vi "Laser_Controller.vi"() -> ()   [LabVIEW 2009]
panel:
  out "Init Error":u32
  out "Intensity (a.u.)":dbl
  out "Close Error Number":u32 format="%.0x"
  in  "PCI Can":bool=TRUE
  out "Excitation":bool
  out "Detector1":bool
  out "Detector2":bool
  out "Intensity (a.u.)":dbl=1.0 format="%.02f"
  in  "Laser(unused)":dbl(slide) scale=0.0..100.0
  in  "?":i16(slide) min=-100 max=100 step=1 scale=-100.0..100.0
  in  "Laser 637 nm (red)":dbl(slide) scale=0.0..100.0
  in  "?":i16(slide) min=-100 max=100 step=1 scale=-100.0..100.0
  in  "Laser 532 nm (green)":dbl(slide) scale=0.0..100.0
  in  "?":i16(slide) min=-100 max=100 step=1 scale=-100.0..100.0
  in  "Laser 470 nm (blue)":dbl(slide) scale=0.0..100.0
  in  "?":i16(slide) min=-100 max=100 step=1 scale=-100.0..100.0
  out "Laser 5 pos.":u16
  out "Laser 6 pos.":u16
  out "Laser 7 pos.":u16
  out "Laser 8 pos.":u16
  out "Laser 4 pos.":u16
  out "Laser 3 pos.":u16
  out "Laser 2 pos.":u16
  out "Laser 1 pos.":u16
  in  "stop":bool
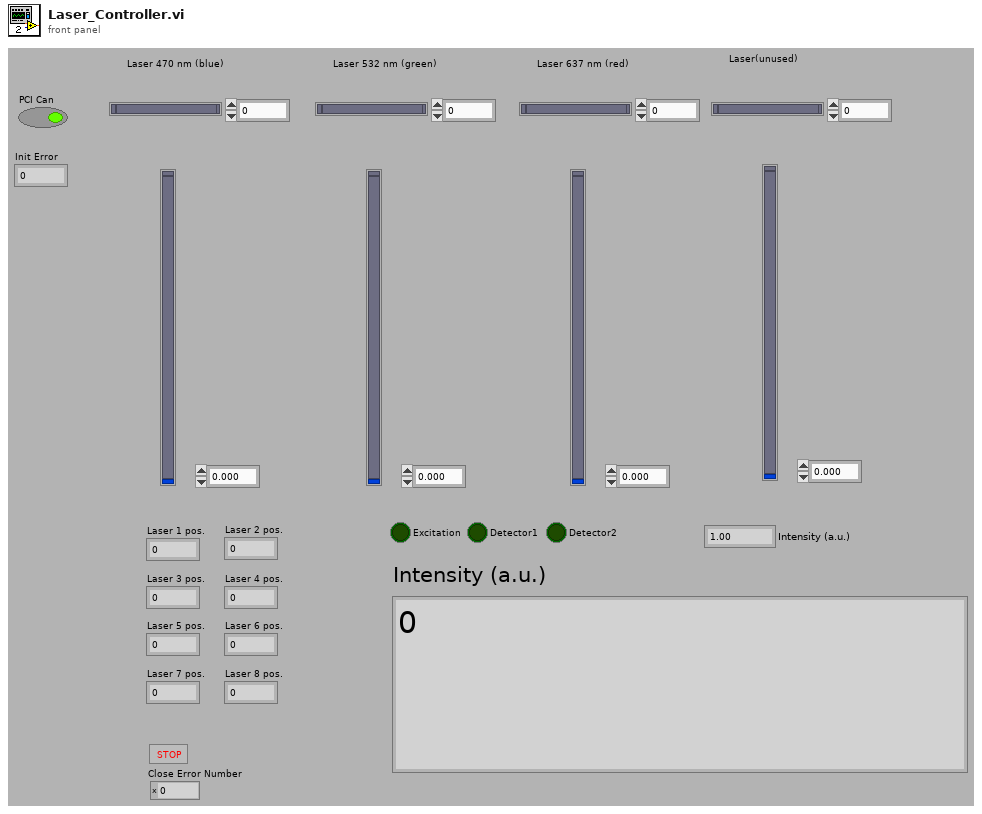
[diagram p1: front panel]
types:
  T1 = enum16{"CAN_Baud_1M", "CAN_BAUD_500K", "CAN_BAUD_250K", "CAN_BAUD_125K", "CAN_BAUD_100K", "CAN_BAUD_50K", "CAN_BAUD_20K", "CAN_BAUD_10K", "CAN_BAUD_5K", "User"}
  T2 = enum8{"STD, NO RTR", "STD,RTR", "XTD, NO RTR", "XTD, RTR"}
  T3 = cluster{"ID":u32, "MSG type":enum8{"STD, NO RTR", "STD,RTR", "XTD, NO RTR", "XTD, RTR"}, "LEN":u8, "DATA":u8[]}
  T4 = cluster{"x":u32, "MSG type":enum8{"STD, NO RTR", "STD,RTR", "XTD, NO RTR", "XTD, RTR"}, "LEN 3":u8, u8[]}
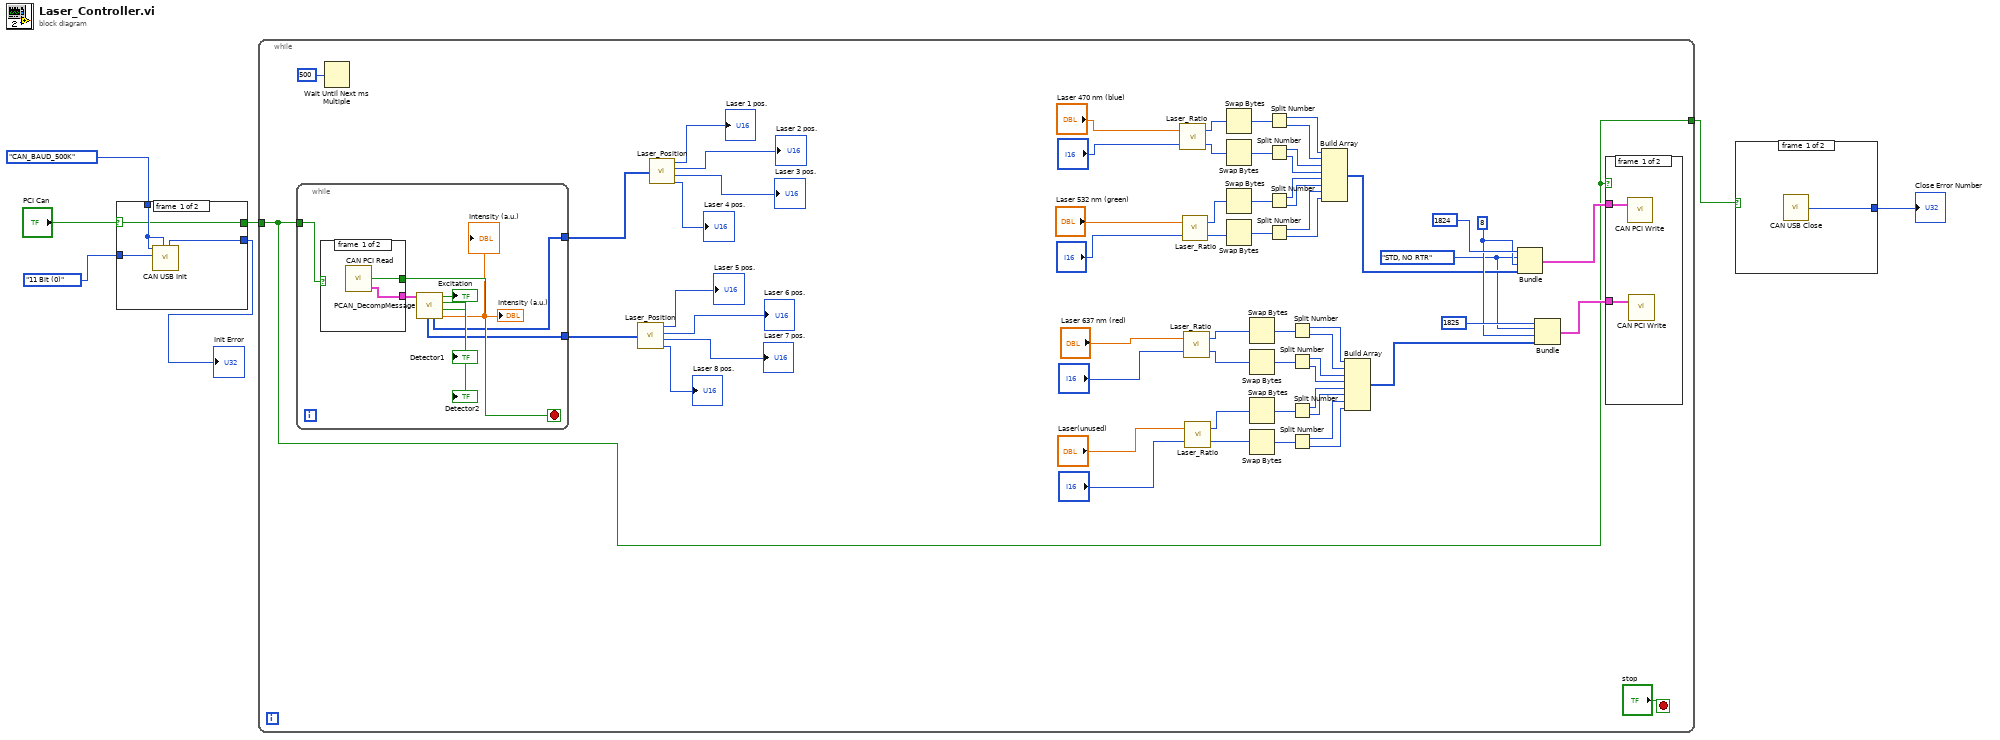
[diagram p0: block diagram]
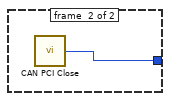
[diagram p2: hidden frame]
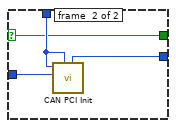
[diagram p3: hidden frame]
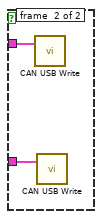
[diagram p4: hidden frame]
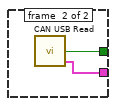
[diagram p5: hidden frame]
diagram:
  n1 = case shown="False" "PCI Can" {
    selector: "PCI Can" -> [w9 w13]
    tunnel: enum16{"11 Bit (0)", "29/11 Bit (1)"}."11 Bit (0)" ("CAN Msg Type") -> [w11 w15]
    tunnel: T1."CAN_BAUD_500K" ("BTR0BTR1") -> [w10 w14]
    tunnel: [w9 w13] -> w4
    tunnel: [w8 w12] -> w1
    frame #0 {
      n2 = call "CAN USB Init.vi"("BTR0BTR1(User)"=w10, "CAN Msg Type"=w11, "BTR0BTR1"=w10) -> ("Error Number"=w8:u32)  [unwired: 6 in, 2 out]
    }
    frame #1 {
      n3 = call "CAN PCI Init.vi"("BTR0BTR1(User)"=w14, "CAN Msg Type"=w15, "BTR0BTR1"=w14) -> ("Error Number"=w12:u32)  [unwired: 6 in, 2 out]
    }
  }
  "Init Error" <- w1
  n4 = while {
    tunnel: w4 -> [w16]
    tunnel: [w16] -> w3
    stop <- "stop" stop-if-true
    w38 = T2."STD, NO RTR" ("MSG type")
    w70 = u8 8 ("LEN 3")
    n5 = while {
      tunnel: w16 -> [w83]
      tunnel: [w82] -> w18
      tunnel: [w81] -> w17
      stop <- w89 stop-if-true
      n6 = case shown="True" w83 {
        tunnel: [w91 w93] -> w89
        tunnel: [w90 w92] -> w88
        frame #0 {
          n7 = call "CAN PCI Read.vi"() -> ("RcvQueueEmpty"=w91:bool, "CAN_Message out"=w90:T3)  [unwired: 1 in, 1 out]
        }
        frame #1 {
          n8 = call "CAN USB Read.vi"() -> ("RcvQueueEmpty"=w93:bool, "CAN_Message out"=w92:T3)  [unwired: 1 in, 1 out]
        }
      }
      n9 = call "PCAN_DecompMessage.vi"("CAN_Message out"=w88) -> ("Intensity (a.u.)"=→"Intensity (a.u.)" →"Intensity (a.u.)":dbl, "Detector2 Shutter Open?"=→"Detector2":bool, "Detector1 Shutter Open?"=→"Detector1":bool, "Excitation Shutter Open?"=→"Excitation":bool, "Laser 1-4"=w82:u8[], "Laser 5-8"=w81:u8[])  [unwired: 5 in]
    }
    n10 = Wait Until Next ms Multiple(millisecond multiple=u32 500) -> ()  [unwired: 1 out]
    n11 = call "Laser_Position.vi"("DATA"=w17) -> ("Laser 1 pos."=→"Laser 5 pos.":u16, "Laser 2 pos."=→"Laser 6 pos.":u16, "Laser 3 pos."=→"Laser 7 pos.":u16, "Laser 4 pos."=→"Laser 8 pos.":u16)
    n12 = call "Laser_Position.vi"("DATA"=w18) -> ("Laser 1 pos."=→"Laser 1 pos.":u16, "Laser 2 pos."=→"Laser 2 pos.":u16, "Laser 3 pos."=→"Laser 3 pos.":u16, "Laser 4 pos."=→"Laser 4 pos.":u16)
    n13 = call "Laser_Ratio.vi"("Numeric 3"="?", "Laser 470 nm (blue)"="Laser 470 nm (blue)") -> ("Numeric"=w51:u16, "Numeric 2"=w52:u16)
    n14 = call "Laser_Ratio.vi"("Numeric 3"="?", "Laser 470 nm (blue)"="Laser 532 nm (green)") -> ("Numeric"=w36:u16, "Numeric 2"=w37:u16)
    n15 = call "Laser_Ratio.vi"("Numeric 3"="?", "Laser 470 nm (blue)"="Laser 637 nm (red)") -> ("Numeric"=w23:u16, "Numeric 2"=w22:u16)
    n16 = call "Laser_Ratio.vi"("Numeric 3"="?", "Laser 470 nm (blue)"="Laser(unused)") -> ("Numeric"=w20:u16, "Numeric 2"=w21:u16)
    n17 = Swap Bytes(anything=w52) -> (byte swapped=w50:u16)
    n18 = Swap Bytes(anything=w51) -> (byte swapped=w49:u16)
    n19 = Swap Bytes(anything=w37) -> (byte swapped=w44:u16)
    n20 = Swap Bytes(anything=w36) -> (byte swapped=w43:u16)
    n21 = Swap Bytes(anything=w22) -> (byte swapped=w35:u16)
    n22 = Swap Bytes(anything=w23) -> (byte swapped=w34:u16)
    n23 = Swap Bytes(anything=w21) -> (byte swapped=w29:u16)
    n24 = Swap Bytes(anything=w20) -> (byte swapped=w28:u16)
    n25 = Split Number(x=w50) -> (hi(x)=w48:u8, lo(x)=w47:u8)
    n26 = Split Number(x=w49) -> (hi(x)=w46:u8, lo(x)=w45:u8)
    n27 = Split Number(x=w44) -> (hi(x)=w42:u8, lo(x)=w39:u8)
    n28 = Split Number(x=w43) -> (hi(x)=w40:u8, lo(x)=w41:u8)
    n29 = Split Number(x=w35) -> (hi(x)=w33:u8, lo(x)=w32:u8)
    n30 = Split Number(x=w34) -> (hi(x)=w31:u8, lo(x)=w30:u8)
    n31 = Split Number(x=w29) -> (hi(x)=w27:u8, lo(x)=w24:u8)
    n32 = Split Number(x=w28) -> (hi(x)=w25:u8, lo(x)=w26:u8)
    n33 = Build Array(w48, w47, w46, w45, w42, w39, w40, w41) -> (w69:u8[])
    n34 = Build Array(w33, w32, w31, w30, w27, w24, w25, w26) -> (w19:u8[])
    n35 = Bundle("x"=u32 1824, "MSG type"=w38, "LEN 3"=w70, w69) -> (w73:T4)  [unwired: 1 in]
    n36 = Bundle("x"=u32 1825, "MSG type"=w38, "LEN 3"=w70, w19) -> (w71:T4)  [unwired: 1 in]
    n37 = case shown="True" w16 {
      tunnel: w73 -> [w78 w80]
      tunnel: w71 -> [w77 w79]
      frame #0 {
        n38 = call "CAN PCI Write.vi"("CAN_Message"=w78) -> ()  [unwired: 2 in, 1 out]
        n39 = call "CAN PCI Write.vi"("CAN_Message"=w77) -> ()  [unwired: 2 in, 1 out]
      }
      frame #1 {
        n40 = call "CAN USB Write.vi"("CAN_Message"=w80) -> ()  [unwired: 2 in, 1 out]
        n41 = call "CAN USB Write.vi"("CAN_Message"=w79) -> ()  [unwired: 2 in, 1 out]
      }
    }
  }
  n42 = case shown="True" w3 {
    tunnel: [w94 w95] -> w2
    frame #0 {
      n43 = call "CAN USB Close.vi"() -> ("Error Number"=w94:u32)  [unwired: 1 in]
    }
    frame #1 {
      n44 = call "CAN PCI Close.vi"() -> ("Error Number"=w95:u32)  [unwired: 1 in]
    }
  }
  "Close Error Number" <- w2
